vi "olimpic_filter (SubVI).vi"(0 "array":dbl[](array[numeric]) format="%#_8g") -> (1 "olimpic_filter":sgl format="%#.2f", 2 "element":dbl format="%#_8g")   [LabVIEW 2017]
panel:
  out "size(s)":i32
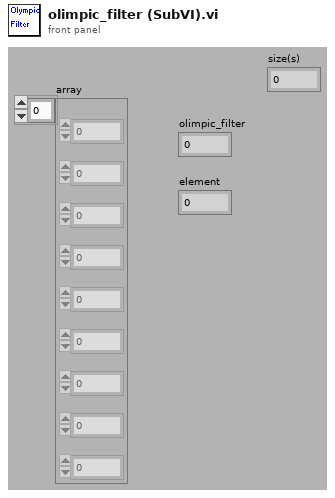
[diagram p1: front panel]
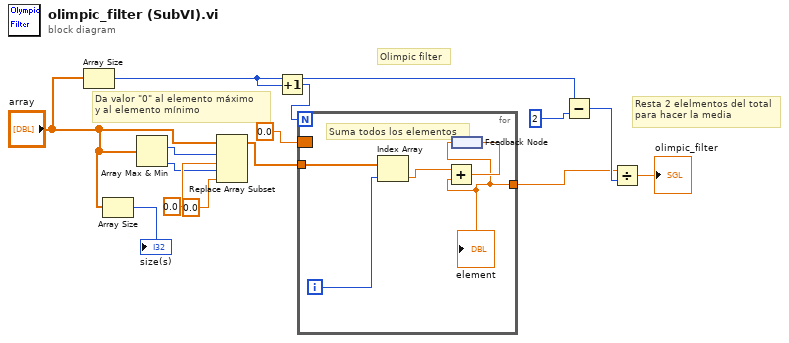
[diagram p0: block diagram]
diagram:
  # "Resta 2 elelmentos del total\npara hacer la media"
  # "Da valor \"0\" al elemento máximo\ny al elemento mínimo"
  # "Olimpic filter"
  n1 = Array Size(array="array") -> (size(s)=w13:i32)
  n2 = Array Size(array="array") -> (size(s)=→"size(s)":i32)
  n3 = Array Max & Min(array="array") -> (max index (indices)=w3:i32, min index (indices)=w4:i32)  [unwired: 2 out]
  n4 = Replace Array Subset(array="array", new element #1=0.0 ("new element/subarray"), index #1=w3, new element #2=0.0 ("new element/subarray"), index #2=w4) -> (w7:dbl[])
  n5 = Increment(x=w13) -> (x+1=w14:i32)
  n6 = for {
    N: w14 -> [_]
    tunnel: w7 -> [w19]
    tunnel: [w15] -> w8
    border: 0.0 -> [_]
    i -> [w18]
    # "Suma todos los elementos"
    n7 = Index Array(array=w19, index=w18) -> (element=w17:dbl)
    n8 = feedback #1() -> (w15:dbl)
    "element" <- w15
    n9 = Add(x=w17, y=w15) -> (x+y=w16:dbl)
    n10 = feedback-in #1(w16) -> ()
  }
  n11 = Subtract(x=w13, y=2) -> (x-y=w10:i32)
  n12 = Divide(x=w8, y=w10) -> (x/y=→"olimpic_filter":dbl)
